vi "Configure Output.vi"(6 "Output Type  (0: Immediate)":u16(ring) items=["Immediate", "Triggered"], 7 "Source Mode  (0: Voltage)":u16(ring) items=["Voltage", "Current"], 8 "error in (no error)":errorcluster, 9 "Compliance  Level (0.1)":dbl=0.1, 10 "Output Level (0)":dbl, 11 "VISA resource name":refnum<visa-resource-name>) -> (0 "error out":errorcluster, 3 "VISA resource name out":refnum<visa-resource-name>)   [LabVIEW 2020, in "Keithley 24XX.lvlib"]
doc: "Configures whether the output is in terms of current or voltage, the amplitude of the output, and compliance settings."
uses:
  Keithley 24XX.lvlib
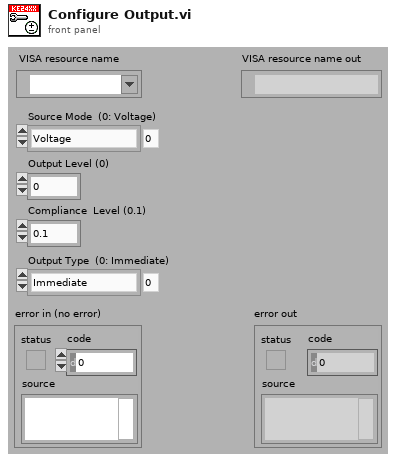
[diagram p1: front panel]
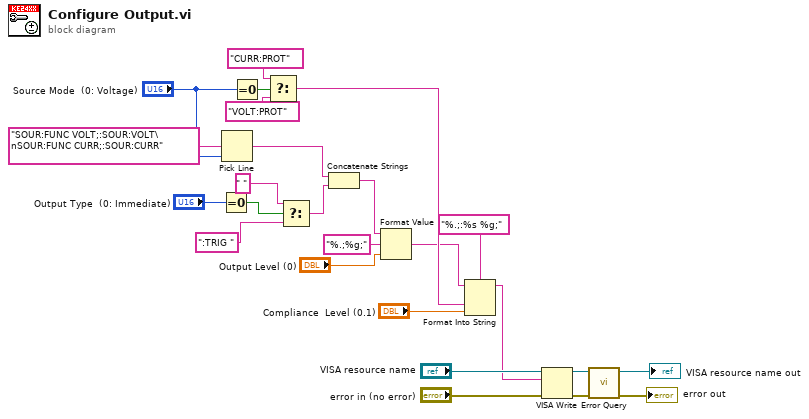
[diagram p0: block diagram]
diagram:
  n1 = Equal To 0?(x="Output Type  (0: Immediate)") -> (x = 0?=w15:bool)
  n2 = Pick Line(multi-line string="SOUR:FUNC VOLT;:SOUR:VOLT\nSOUR:FUNC CURR;:SOUR:CURR", line index="Source Mode  (0: Voltage)") -> (output string=w11:string)  [unwired: 1 in]
  n3 = Equal To 0?(x="Source Mode  (0: Voltage)") -> (x = 0?=w8:bool)
  n4 = Select(t="CURR:PROT", s=w8, f="VOLT:PROT") -> (s? t:f=w5:string)
  n5 = Select(t=" ", s=w15, f=":TRIG ") -> (s? t:f=w12:string)
  n6 = Concatenate Strings(w11, w12) -> (w10:string)
  n7 = Format Value(string ("")=w10, format string="%.;%g;", value (0)="Output Level (0)") -> (output string=w3:string)
  n8 = Format Into String(format string="%.;:%s %g;", initial string=w3, w5, "Compliance  Level (0.1)") -> (resulting string=w2:string)  [unwired: 1 in, 1 out]
  n9 = VISA Write(VISA resource name="VISA resource name", write buffer=w2, error in (no error)="error in (no error)") -> (VISA resource name out=w21:refnum<visa-resource-name>, error out=w20:errorcluster)  [unwired: 1 out]
  n10 = call "Error Query.vi"("error in (no error)"=w20, "VISA resource name"=w21) -> ("error out"=→"error out":errorcluster, "VISA resource name out"=→"VISA resource name out":refnum<visa-resource-name>)  [unwired: 6 in, 2 out]
